vi "Establish Serial Coms.vi"(8 "error in (no error)":errorcluster) -> (0 "error IO":errorcluster, 1 "abort":bool, 2 "Control Board":refnum<visa-resource-name>)   [LabVIEW 2022 SP3]
uses:
  <vilib>/Instr/_visa.llb/VISA Configure Serial Port (Instr).vi
panel:
  in  "abort":bool
  in  "stop":bool
  out "Instructional Message":string
  out "Unsuccesful Attempts to connect":i32
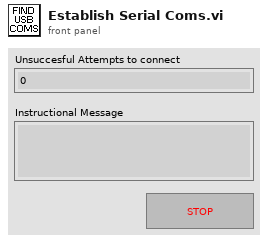
[diagram p1: front panel]
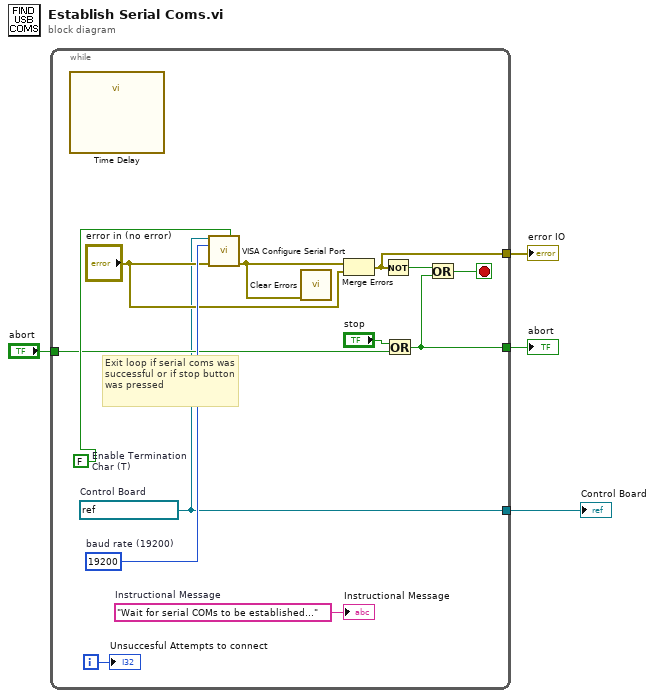
[diagram p0: block diagram]
diagram:
  n1 = while {
    tunnel: [w9] -> w4
    tunnel: [w5] -> w3
    tunnel: "abort" -> [w8]
    tunnel: [w7] -> w1
    i -> [w13]
    stop <- w11 stop-if-true
    w12 = "Wait for serial COMs to be established..."  # Instructional Message
    w17 = FALSE  # Enable Termination Char (T)
    w16 = u32 19200  # baud rate (19200)
    w7 = refnum<visa-resource-name> "ControlBoard"  # Control Board
    # "Exit loop if serial coms was successful or if stop button was pressed"
    n2 = call "Time Delay"() -> ()  [unwired: 11 in, 1 out]
    n3 = call-poly "VISA Configure Serial Port"("VISA resource name"=w7, "Enable Termination\nChar (T)"=w17, "baud rate (9600)"=w16, "error in (no error)"="error in (no error)") -> ("error out"=w6:errorcluster)  [unwired: 10 in, 1 out]
    n4 = call <vilib>:"Clear Errors.vi"("error in (no error)"=w6) -> ()  [unwired: 5 in, 2 out]
    n5 = Merge Errors(w6, "error in (no error)") -> (w5:errorcluster)
    n6 = Not(x=w5) -> (.not. x?=w14:bool)
    n7 = Or(x="stop", y=w8) -> (x .or. y?=w9:bool)
    n8 = Or(x=w14, y=w9) -> (x .or. y?=w11:bool)
    "Unsuccesful Attempts to connect" <- w13
    "Instructional Message" <- w12
  }
  "Control Board" <- w1
  "abort" <- w4
  "error IO" <- w3
